vi "StopSignal-IsValid.vi"(8 "error in (no error)":errorcluster, 9 "timeout in ms (0)":i32, 11 "StopSignal":T1) -> (0 "error out":errorcluster, 1 "valid?":bool, 3 "StopSignal(dup)":T1)   [LabVIEW 2017, in "StopSignal.lvlib"]
uses:
  StopSignal.lvlib
  Typedef/StopSignal.ctl
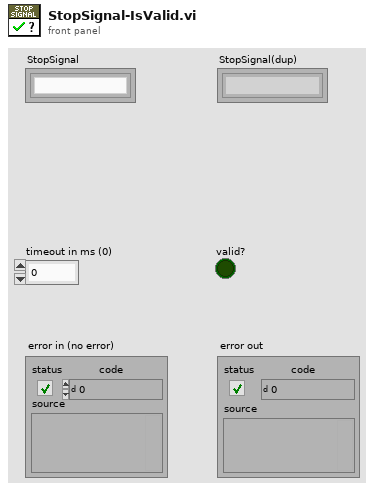
[diagram p1: front panel]
types:
  T1 = typedef "StopSignal.lvlib/StopSignal.ctl" = refnum<k1>
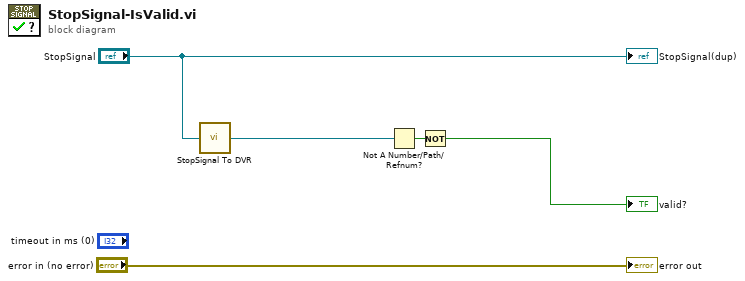
[diagram p0: block diagram]
diagram:
  n1 = call "StopSignal To DVR.vi"("Refnum in"="StopSignal") -> ("Data Value Reference out"=w3:refnum<data-value>)
  n2 = Not A Number/Path/Refnum?(number/path/refnum=w3) -> (NaN/Path/Refnum?=w2:bool)
  n3 = Not(x=w2) -> (.not. x?=→"valid?":bool)
  "error out" <- "error in (no error)"
  "StopSignal(dup)" <- "StopSignal"
